vi "Convert OLE Color to labview Color.vi"(1 "color in":u32(colorbox)=16711680 caption="颜色输入") -> (0 "color out":u32(colorbox)=255 caption="颜色输出")   [LabVIEW 2011]
doc: "使LabVIEW颜色转换为ActiveX的颜色，或进行相反操作。"
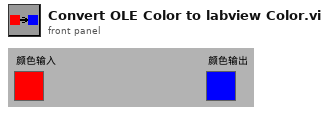
[diagram p1: front panel]
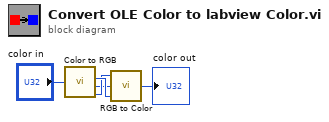
[diagram p0: block diagram]
diagram:
  n1 = call <vilib>:"Color to RGB.vi"("Color"="color in") -> ("R"=w3:u8, "G"=w1:u8, "B"=w2:u8)  [unwired: 1 out]
  n2 = call <vilib>:"RGB to Color.vi"("B"=w3, "G"=w1, "R"=w2) -> ("Color"=→"color out":u32)
